vi "create.volume.index.vi"(8 "error in (no error)":errorcluster, 9 "output filepath":path=path "D:/Comics/data/key_maps/volumes.json", 10 "Issue Path":path=path "D:/Comics/data/cv_issues", 11 "Volume Path":path=path "D:/Comics/data/cv_volumes") -> (0 "error out":errorcluster)   [LabVIEW 2024]
uses:
  definitions/volume.index--cluster.ctl
  definitions/comicvine_issue.generic_credit.ctl
  <vilib>/addons/_JKI.lib/Serialization/JSON/JKI JSON Serialization.lvlib
panel:
  out "current volume":string
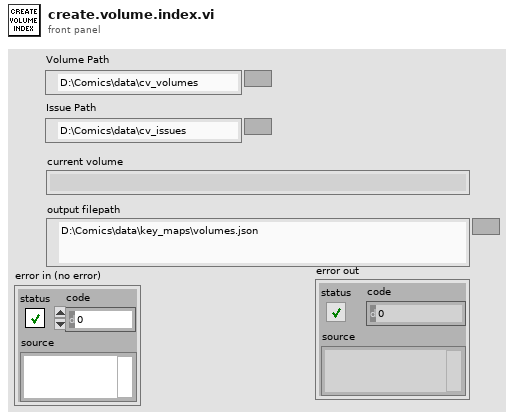
[diagram p1: front panel]
types:
  T1 = cluster{"volume":string, "characters":cluster{"id":i32, "name":string, "count":i32}[], "teams":cluster{"id":i32, "name":string, "count":i32}[], "start":timestamp, "end":timestamp, "count_of_issues":i32}
  T2 = typedef "comicvine_issue.generic_credit.ctl" = cluster{"id":i32, "name":string}
  T3 = map{string, cluster{"chars":map{T2, i32}, "teams":map{T2, i32}, "start":timestamp, "end":timestamp, "count_of_issues":i32}}
  T4 = typedef "volume.index--cluster.ctl" = cluster{"volume_map":cluster{"volume":string, "characters":cluster{"id":i32, "name":string, "count":i32}[], "teams":cluster{"id":i32, "name":string, "count":i32}[], "start_date":timestamp, "end_date":timestamp, "count_of_issues":i32}[]}
  T5 = cluster{"chars":map{T2, i32}, "teams":map{T2, i32}, "start":timestamp, "end":timestamp, "count_of_issues":i32}
  T6 = typedef "local_volume.ctl" = cluster{"id":i32, "name":string, "sortable_name":string, "aliases":string[], "description":string, "site_detail_url":string, "count_of_issues":i32, "start_year":i32, "publisher_id":i32, "issue_ids":i32[], "date_last_updated":timestamp, "volume":i32, "cv_id":string}
  T7 = typedef "local_issue.ctl" = cluster{"cover_date":timestamp, "id":i32, "cv_id":string, "name":string, "sortable_name":string, "issue_number":string, "deck":string, "description":string, "volume":T2, "store_date":timestamp, "date_last_updated":timestamp, "site_detail_url":string, "cover_url":string, "associated_images":T8[], "characters":T2[], "concepts":T2[], "creators":T9[], "storyArcs":T2[], "teams":T2[]}
  T8 = typedef "comicvine_issue.associated_image.ctl" = cluster{"original_url":string, "id":i32}
  T9 = typedef "comicvine_issue.person_credit.ctl" = cluster{"id":i32, "name":string, "role":string}
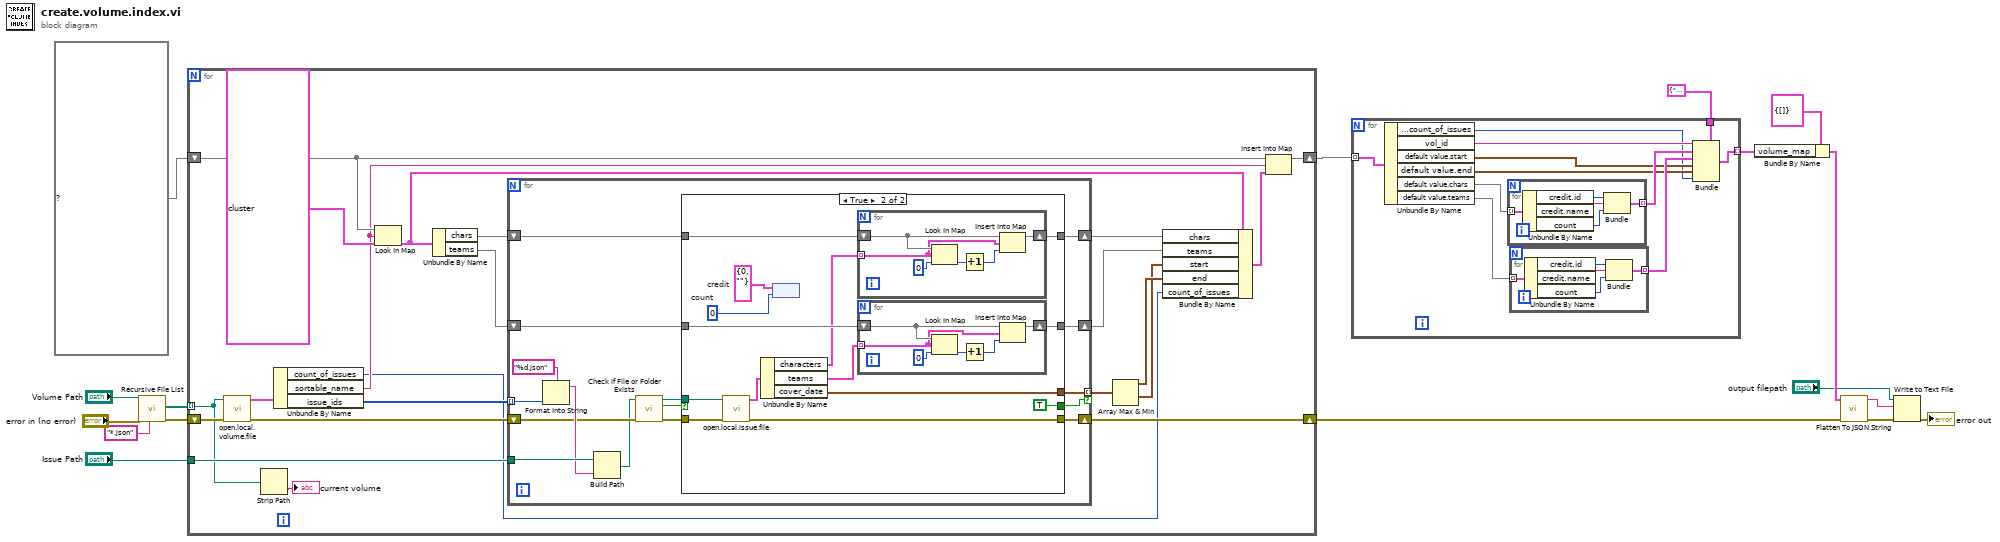
[diagram p0: block diagram]
diagram:
  n1 = call <vilib>:"Recursive File List.vi"("pattern"="*.json", "error in (no error)"="error in (no error)", "Folder Path"="Volume Path") -> ("error out"=w15:errorcluster, "All Files in Dir"=w14:path[])  [unwired: 4 in, 3 out]
  n2 = for {
    shift-right: [w33] -> w8
    shift-left: w15 -> [w39]
    tunnel: w14 -> [w32] mode=indexing
    tunnel: "Issue Path" -> [w36]
    shift-right: [w34] -> w12
    shift-left: T3 {} ("map") -> [w30]
    n3 = call "open.local.volume.file.vi"("error in (no error)"=w39, "volume json"=w32) -> ("error out"=w35:errorcluster, "volume"=w38:T6)  [unwired: 8 in]
    n4 = Strip Path(path=w32) -> (name=→"current volume":string)  [unwired: 1 out]
    n5 = Unbundle By Name(w38) -> ("count_of_issues"=w18:i32, "sortable_name"=w22:string, "issue_ids"=w37:i32[])
    n6 = Look In Map(map=w30, key=w22, default value=T5 {"chars"={}, "teams"={}, "start"=timestamp(0 s since 1904-01-01), "end"=timestamp(0 s since 1904-01-01), "count_of_issues"=0}) -> (value=w26:T5)  [unwired: 1 out]
    n7 = Unbundle By Name(w26) -> ("chars"=w27:map{T2, i32}, "teams"=w28:map{T2, i32})
    n8 = for {
      tunnel: w37 -> [w54] mode=indexing
      tunnel: w36 -> [w53]
      shift-right: [w44] -> w33
      shift-left: w35 -> [w51]
      shift-right: [w45] -> w24
      shift-left: w28 -> [w46]
      shift-right: [w42] -> w25
      shift-left: w27 -> [w43]
      tunnel: [w41] -> w21 mode=indexing if=w40
      n9 = Format Into String(format string="%d.json", w54) -> (resulting string=w52:string)  [unwired: 2 in, 1 out]
      n10 = Build Path(base path=w53, name or relative path=w52) -> (appended path=w50:path)
      n11 = call <vilib>:"Check if File or Folder Exists.vi"("error in (no error)"=w51, "path"=w50) -> ("error out"=w47:errorcluster, "file or folder exists?"=w49:bool, "dup path"=w48:path)  [unwired: 7 in]
      n12 = case shown="True" w49 {
        tunnel: w48 -> [_ w72]
        tunnel: w47 -> [w57 w71]
        tunnel: w46 -> [w58 w69]
        tunnel: [w58 w68] -> w45
        tunnel: [w57 w67] -> w44
        tunnel: w43 -> [w56 w66]
        tunnel: [w56 w64] -> w42
        tunnel: [_ w60] -> w41
        tunnel: [_ TRUE] -> w40
        frame False {
        }
        frame True {
          w61 = 0  # count
          w62 = T2 {"id"=0, "name"=""}  # credit
          n13 = call "open.local.issue.file.vi"("error in (no error)"=w71, "volume json"=w72) -> ("error out"=w67:errorcluster, "issue"=w70:T7)  [unwired: 8 in]
          n14 = Unbundle By Name(w70) -> ("characters"=w63:T2[], "teams"=w65:T2[], "cover_date"=w60:timestamp)
          n15 = node(w62, w61) -> ()  [unwired: 1 out]
          n16 = for {
            tunnel: w63 -> [w73] mode=indexing
            shift-right: [w74] -> w64
            shift-left: w66 -> [w75]
            n17 = Look In Map(map=w75, key=w73, default value=0) -> (value=w77:i32)  [unwired: 1 out]
            n18 = Increment(x=w77) -> (x+1=w76:i32)
            n19 = Insert Into Map(map in=w75, key=w73, value=w76) -> (map out=w74:map{T2, i32})  [unwired: 2 out]
          }
          n20 = for {
            tunnel: w65 -> [w79] mode=indexing
            shift-right: [w80] -> w68
            shift-left: w69 -> [w81]
            n21 = Look In Map(map=w81, key=w79, default value=0) -> (value=w83:i32)  [unwired: 1 out]
            n22 = Increment(x=w83) -> (x+1=w82:i32)
            n23 = Insert Into Map(map in=w81, key=w79, value=w82) -> (map out=w80:map{T2, i32})  [unwired: 2 out]
          }
        }
      }
    }
    n24 = Array Max & Min(array=w21) -> (max value=w20:timestamp, min value=w19:timestamp)  [unwired: 2 out]
    n25 = Bundle By Name(cluster=w26, "chars"=w25, "teams"=w24, "start"=w19, "end"=w20, "count_of_issues"=w18) -> (w23:T5)
    n26 = Insert Into Map(map in=w30, key=w22, value=w23) -> (map out=w34:T3)  [unwired: 2 out]
  }
  n27 = for {
    tunnel: w12 -> [w95] mode=indexing
    tunnel: T1 {"volume"="", "characters"=[], "teams"=[], "start"=timestamp(0 s since 1904-01-01), "end"=timestamp(0 s since 1904-01-01), "count_of_issues"=0} ("output cluster") -> [w93]
    tunnel: [w92] -> w10 mode=indexing
    n28 = Unbundle By Name(w95) -> ("default value.count_of_issues"=w85:i32, "vol_id"=w94:string, "default value.start"=w87:timestamp, "default value.end"=w86:timestamp, "default value.chars"=w88:map{T2, i32}, "default value.teams"=w91:map{T2, i32})
    n29 = for {
      tunnel: w88 -> [w105] mode=indexing
      tunnel: [w102] -> w90 mode=indexing
      n30 = Unbundle By Name(w105) -> ("credit.id"=w104:i32, "credit.name"=w103:string, "count"=w101:i32)
      n31 = Bundle("id"=w104, "name"=w103, "count"=w101) -> (w102:cluster{"id":i32, "name":string, "count":i32})  [unwired: 1 in]
    }
    n32 = for {
      tunnel: w91 -> [w100] mode=indexing
      tunnel: [w97] -> w89 mode=indexing
      n33 = Unbundle By Name(w100) -> ("credit.id"=w99:i32, "credit.name"=w98:string, "count"=w96:i32)
      n34 = Bundle("id"=w99, "name"=w98, "count"=w96) -> (w97:cluster{"id":i32, "name":string, "count":i32})  [unwired: 1 in]
    }
    n35 = Bundle(cluster=w93, "volume"=w94, "characters"=w90, "teams"=w89, "start"=w87, "end"=w86, "count_of_issues"=w85) -> (w92:T1)
  }
  n36 = Bundle By Name(cluster=T4 {"volume_map"=[]}, "volume_map"=w10) -> (w9:T4)
  n37 = call <vilib>:"Flatten To JSON String.vi"("error in"=w8, "Variant"=w9) -> ("error out"=w7:errorcluster, "JSON String"=w6:string)  [unwired: 8 in]
  n38 = Write to Text File(file (use dialog)="output filepath", text=w6, error in=w7) -> (error out=→"error out":errorcluster)  [unwired: 1 in, 2 out]
